vi "NT Read Name Cache.vi"(11 "Name":string) -> (2 "Success":bool, 3 "Field Value Out":T1)   [LabVIEW 2017]
uses:
  <vilib>/Rock Robotics/Network Tables/Field Data.ctl
  <vilib>/Rock Robotics/Network Tables/Field Type.ctl
  <vilib>/Rock Robotics/Network Tables/Sequence.ctl
  <vilib>/Rock Robotics/Network Tables/Make Table Operation.ctl
  <vilib>/Rock Robotics/Network Tables/NT Globals.vi
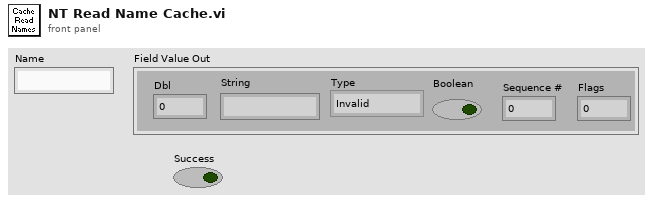
[diagram p1: front panel]
types:
  T1 = typedef "Field Data.ctl" = cluster{"Dbl":dbl, "String":string, "Type":T2, "Boolean":bool, "Sequence #":T3, "Flags":u8}
  T2 = typedef "Field Type.ctl" = enum8{"Invalid", "Bool", "Numeric", "String", "Raw", "Boolean Array", "Numeric Array", "String Array", "RPC"}
  T3 = typedef "Sequence.ctl" = u16
  T4 = typedef "Make Table Operation.ctl" = enum16{"Get or Add Field", "Get Field or Add Temp", "Replace Temp ID", "Get Field ID - No Add", "Get Table Field IDs", "Get Field ID Info", "Move Field to Temp", "Validate", "Remove Field", "Remove All"}
  T5 = typedef "Field ID.ctl" = i32
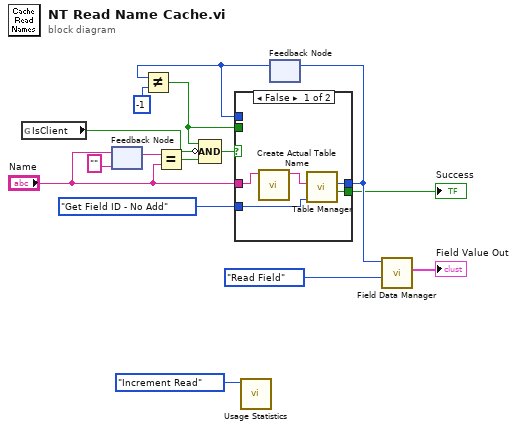
[diagram p0: block diagram]
diagram:
  n1 = global read "NT Globals.vi" "IsClient"() -> (w2:bool)
  n2 = feedback #1("" ("Name")) -> (w12:string)
  n3 = feedback-in #1("Name") -> ()
  n4 = Equal?(x=w12, y="Name") -> (x = y?=w13:bool)
  n5 = call <vilib>:"Usage Statistics.vi"("Operation"=enum16{"Increment Read", "Increment Write"}."Increment Read") -> ()  [unwired: 11 in]
  n6 = feedback #2() -> (w4:T5)  [unwired: 1 in]
  n7 = Not Equal?(x=w4, y=-1) -> (x != y?=w3:bool)
  n8 = Compound Arithmetic op=AND(w3, invert w2, w13) -> (w14:bool)
  n9 = case shown="False" w14 {
    tunnel: "Name" -> [w16 _]
    tunnel: [w20 w22] -> w9
    tunnel: [w19 w21] -> w8
    tunnel: Make_Table_Operation."Get Field ID - No Add" ("Operation") -> [w18 _]
    tunnel: w4 -> [_ w22]
    tunnel: w3 -> [_ w21]
    frame False {
      n10 = call <vilib>:"Create Actual Table Name.vi"("Name or Path"=w16) -> ("Absolute Path"=w17:string)  [unwired: 10 in]
      n11 = call <vilib>:"Table Manager.vi"("Operation"=w18, "Entry Name"=w17) -> ("Success"=w19:bool, "Entry ID"=w20:T5)  [unwired: 6 in, 2 out]
    }
    frame True {
    }
  }
  "Success" <- w8
  n12 = feedback-in #2(w9) -> ()
  n13 = call <vilib>:"Field Data Manager.vi"("Operation"=enum16{"Update Field", "Read Field"}."Read Field", "Field ID"=w9) -> ("Field Value Out"=→"Field Value Out":T1)  [unwired: 8 in, 1 out]
